vi "Write N.vi"(10 "N":i32=5000, 11 "OscillationDetector in":refnum<class "OscillationDetector.lvclass">) -> (3 "OscillationDetector out":refnum<class "OscillationDetector.lvclass">)   [LabVIEW 2019, in "OscillationDetector.lvclass"]
uses:
  OscillationDetector.lvclass
  OscillationDetector.lvclass/OscillationDetector.ctl
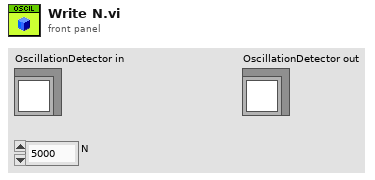
[diagram p1: front panel]
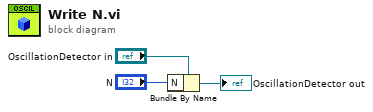
[diagram p0: block diagram]
diagram:
  n1 = Bundle By Name(cluster="OscillationDetector in", "N"="N") -> (→"OscillationDetector out":refnum<class "OscillationDetector.lvclass">)
